vi "Match Regular Expression.vi"() -> ()   [LabVIEW 2016]
uses:
  <vilib>/regexp/Match Regular Expression.xnode
panel:
  out "error out":errorcluster
  out "offset past match":i32
  out "after match":string
  out "whole match":string
  out "before match":string
  in  "multiline? (F)":bool
  in  "ignore case? (F)":bool
  in  "error in":errorcluster
  in  "offset (0)":i32
  in  "regular expression":string
  in  "input string":string
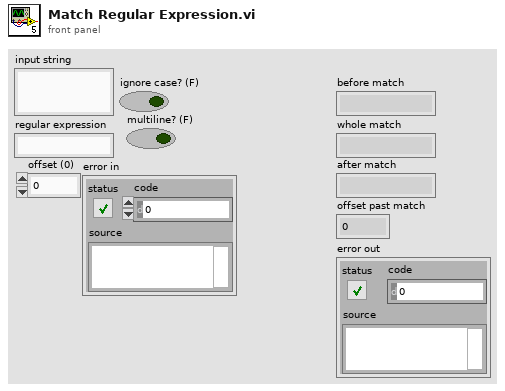
[diagram p1: front panel]
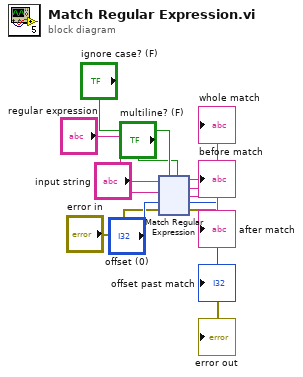
[diagram p0: block diagram]
diagram:
  n1 = xnode "Match Regular Expression"("input string"="input string", "regular expression"="regular expression", "offset (0)"="offset (0)", "error in"="error in", "ignore case? (F)"="ignore case? (F)", "multiline? (F)"="multiline? (F)") -> ("before match"=→"before match":string, "whole match"=→"whole match":string, "after match"=→"after match":string, "offset past match"=→"offset past match":i32, "error out"=→"error out":errorcluster)
